vi "PrependRows.vi"   [LabVIEW 2009]
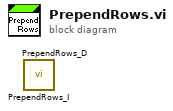
[diagram p0: block diagram]
diagram:
  n1 = call "PrependRows_I.vi"() -> ()  [unwired: 11 in, 1 out]
  n2 = call "PrependRows_D.vi"() -> ()  [unwired: 11 in, 1 out]
